vi "Control_Channel_Status.vi"() -> ()   [LabVIEW 2022 SP3]
uses:
  Sub VIs/ADAM Controls/Channel_State.ctl
  Sub VIs/ADAM Controls/Channel_names.ctl
  ADAM Server/ADAM_Global.vi
  Anemometry/Anemometry Sub Vis/Globals/Preference_global.vi
panel:
  out "Message":string
  out "List of Addresses":string[](array[string])
  in  "Address":u16(ring) items=["Show All", "0", "1", "502"]
  out "List of Ports":string[](array[string])
  in  "Port Names":u16(ring) items=["Show All", "", "LabVIEW", "10.244.4.15:502", "10.244.5.42"]
  out "Turn On?":bool
  in  "Turn Channel Off?":bool
  in  "stop":bool
  out "Ch State":T1
  in  "Turn Channels On?":bool
  in  "Selected Channels to Edit":i32[](listbox)
  in  "Search Charcters":string
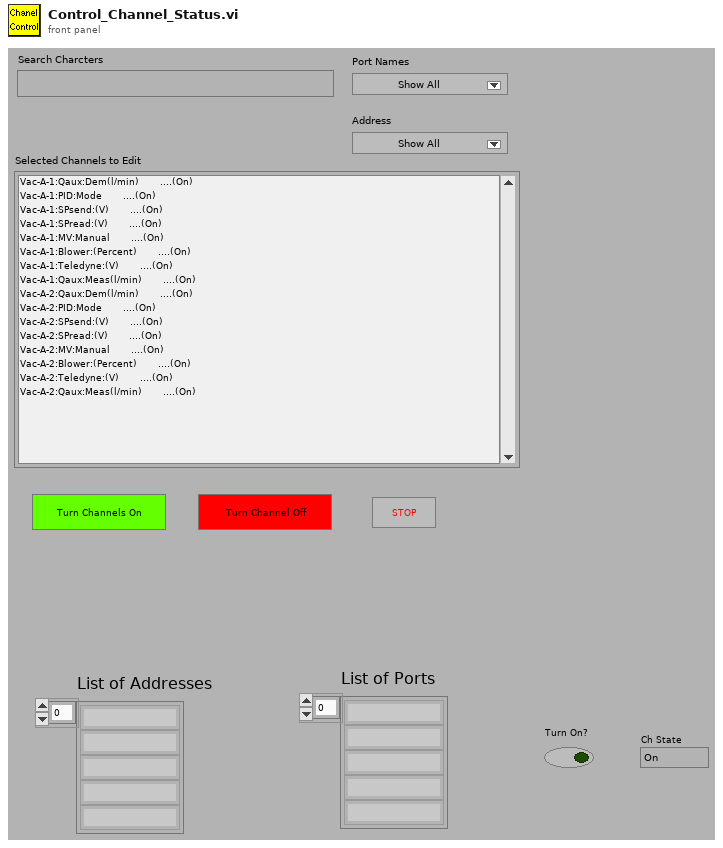
[diagram p1: front panel]
types:
  T1 = typedef "Channel_State.ctl" = enum16{"On", "Off", "Always On", "Always Off"}
  T2 = typedef "Channel_names.ctl" = enum16{"Active Only", "Active + Off", "All Channels", "Changeable Only", "Always Off", "Always On", "Always Off or On"}
  T3 = typedef "Server_Comms.ctl" = enum16{"Do Not Link To Server", "Server Link Healthy"}
  T4 = typedef "Ch_description_ADAM.ctl" = cluster{"Ch Name":string, "Type":T5, "Function":T6, "Ch State":T1, "Calibration type":T7, "A":dbl, "B":dbl, "C":dbl, "D":dbl, "Comments":string, "Address":T8, "String":string, "Duty":u16}
  T5 = typedef "Module_type_ADAM.ctl" = string
  T6 = typedef "Function_ADAM.ctl" = enum16{"Analogue Input", "Digital Input", "Event counter", "Event rate", "Analogue Output", "Digital Output", "Relay Output"}
  T7 = typedef "Calib_type_ADAM.ctl" = string
  T8 = typedef "Address.ctl" = cluster{"Main":i32, "Ch.":i32, "Sub":i32, "Port Name":string}
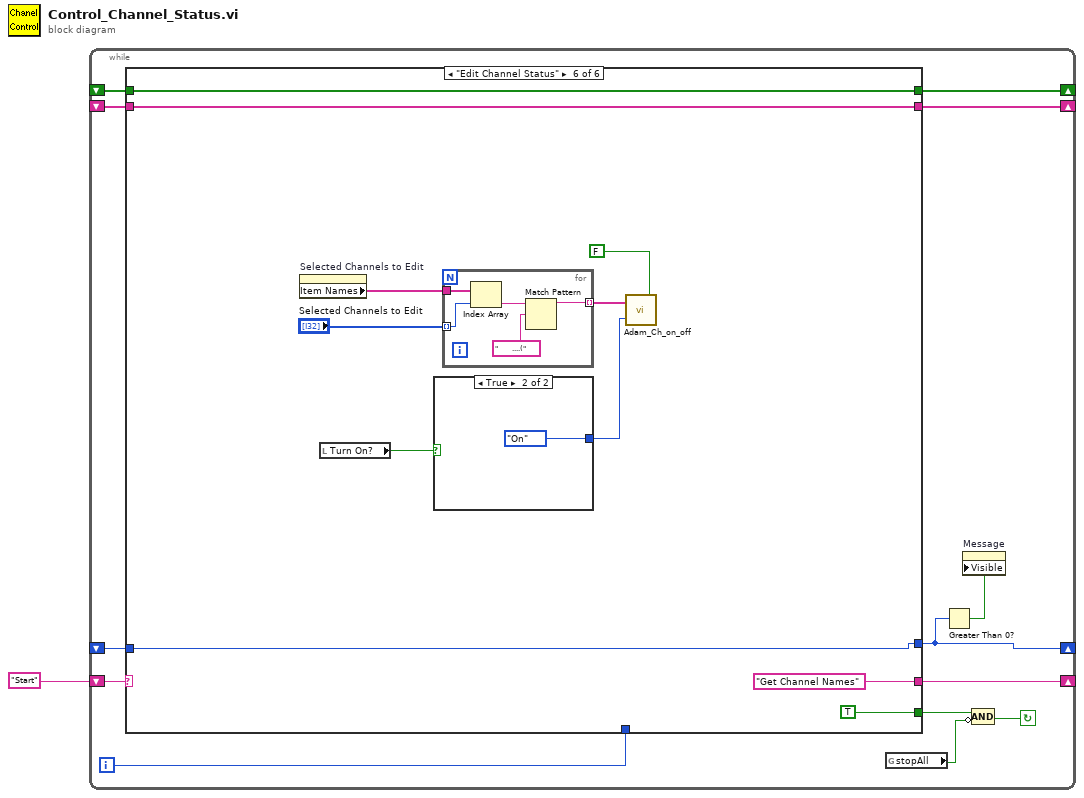
[diagram p0: block diagram]
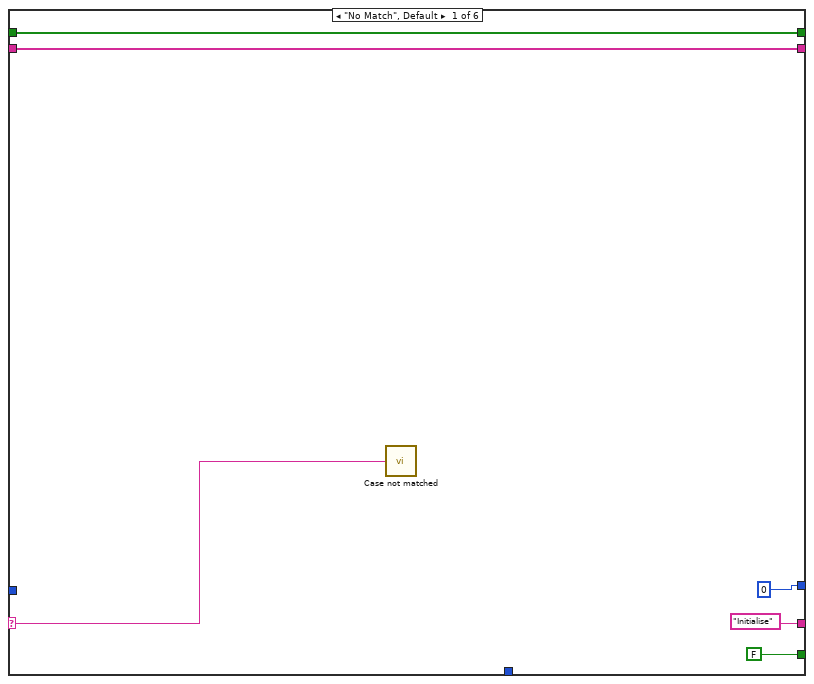
[diagram p2: hidden frame]
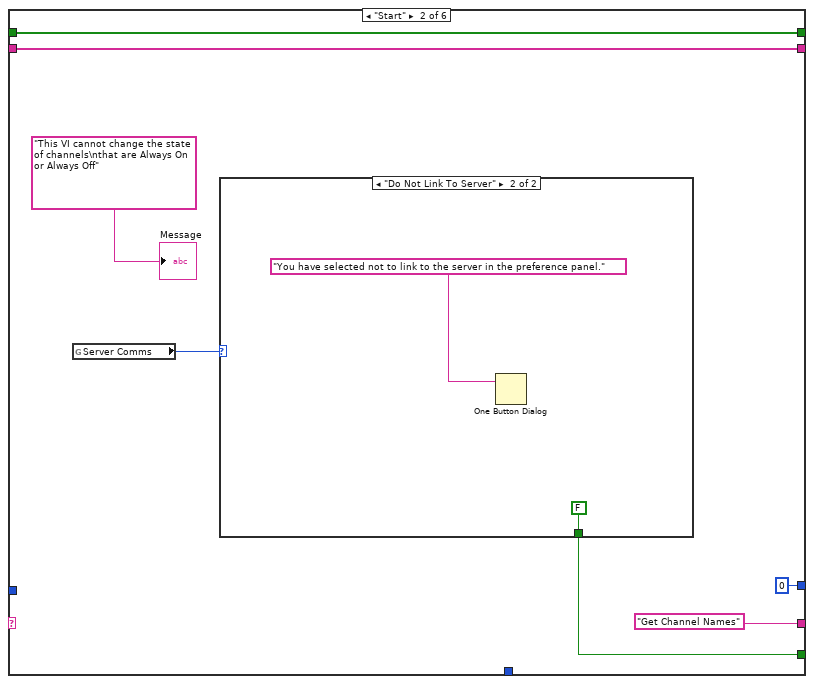
[diagram p3: hidden frame]
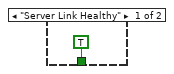
[diagram p4: hidden frame]
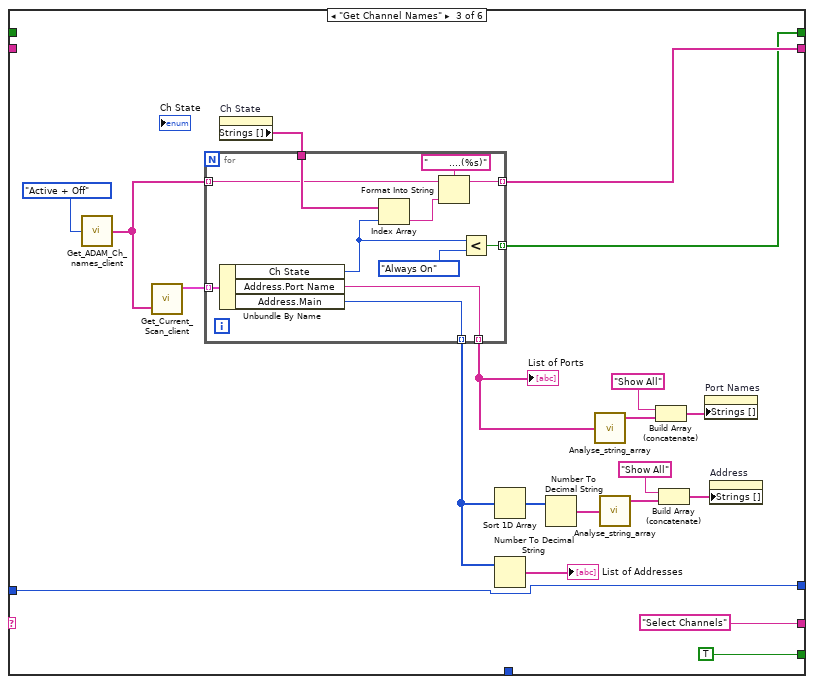
[diagram p5: hidden frame]
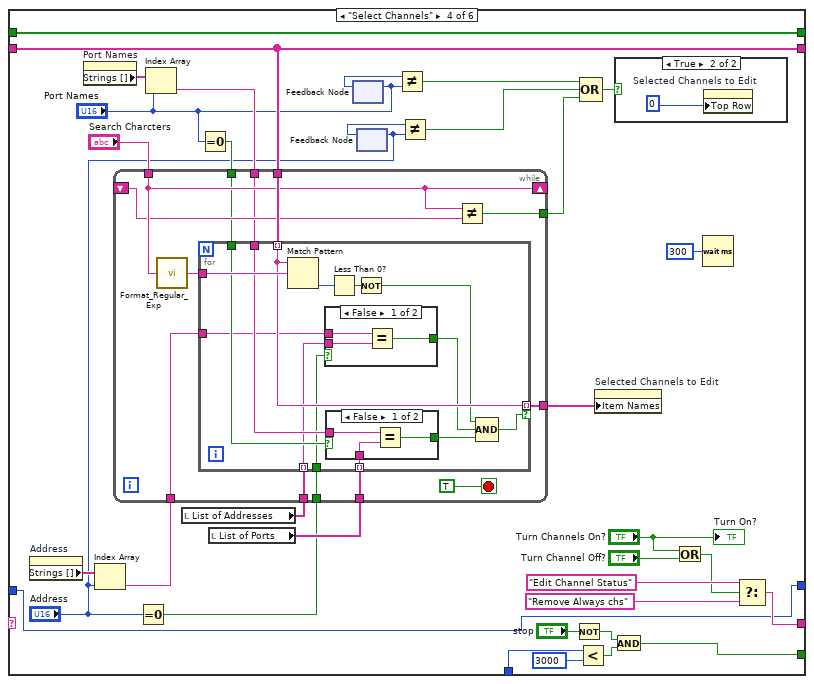
[diagram p6: hidden frame]
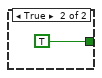
[diagram p8: hidden frame]
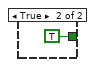
[diagram p9: hidden frame]
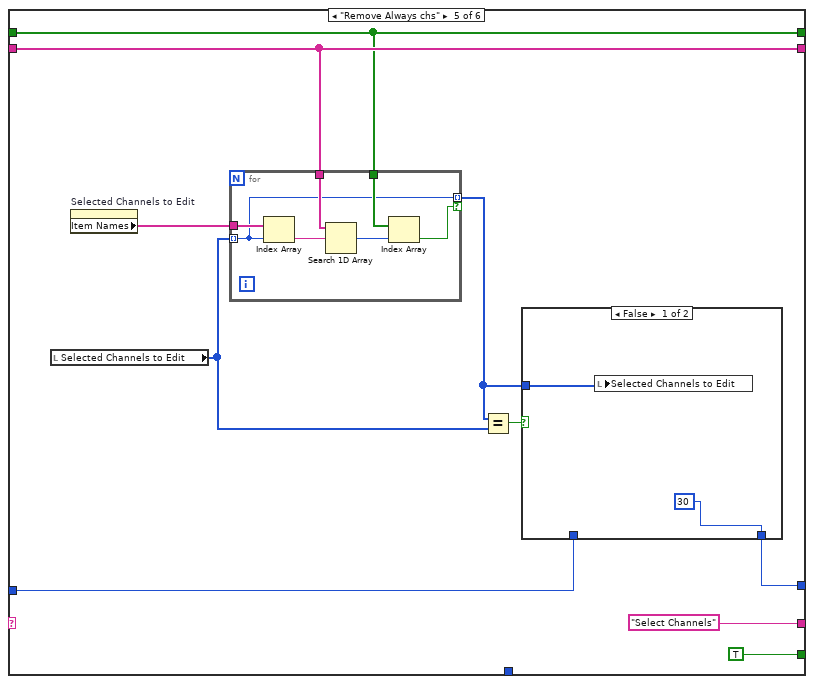
[diagram p10: hidden frame]
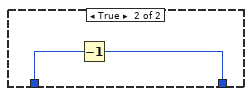
[diagram p11: hidden frame]
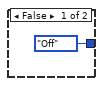
[diagram p12: hidden frame]
diagram:
  n1 = while {
    shift-left: "Start" -> [w13]
    shift-right: [w14] -> _
    shift-right: [w12] -> _
    shift-left: _ -> [w11]
    shift-right: [w9] -> _
    shift-left: _ -> [w8]
    shift-right: [w6] -> _
    shift-left: _ -> [w7]
    i -> [w10]
    stop <- w4 continue-if-true
    n2 = case shown="\"Edit Channel Status\"" w13 {
      selector: w13 -> [w16 _ _ _ _ _]
      tunnel: [FALSE w25 TRUE w82 TRUE TRUE] -> w3
      tunnel: ["Initialise" "Get Channel Names" "Select Channels" w92 "Select Channels" "Get Channel Names"] -> w14
      tunnel: [w18 w24 w44 w90 w138 w163] -> w12
      tunnel: w11 -> [w18 w24 _ w90 w138 w163]
      tunnel: w10 -> [_ _ _ w81 _ _]
      tunnel: [w17 w23 w32 w65 w137 w155] -> w9
      tunnel: w8 -> [w17 w23 _ w65 w137 w155]
      tunnel: [0 0 w31 w62 w133 w154] -> w6
      tunnel: w7 -> [_ _ w31 w62 w132 w154]
      frame "No Match", Default {
        n3 = call "Case not matched.vi"("Case Name not Matched"=w16) -> ()
      }
      frame "Start" {
        n4 = global read "Preference_global.vi" "Server Comms"() -> (w26:T3)
        n5 = case shown="\"Do Not Link To Server\"" w26 {
          tunnel: [TRUE FALSE] -> w25
          frame "Server Link Healthy" {
          }
          frame "Do Not Link To Server" {
            n6 = One Button Dialog(message="You have selected not to link to the server in the preference panel.") -> ()  [unwired: 2 out]
          }
        }
        "Message" <- "This VI cannot change the state of channels\nthat are Always On or Always Off"
      }
      frame "Get Channel Names" {
        n7 = call "Get_ADAM_Ch_names_client.vi"("Channel names set"=Channel_names."Active + Off") -> ("Ch names"=w45:string[])
        n8 = call "Get_Current_Scan_client.vi"("multipleChannels"=w45) -> ("Ch Description Array"=w47:T4[])  [unwired: 1 in, 3 out]
        n9 = property on="Ch State" class="Enum (strict)"() -> ("Strings []"=w46:string[])  [unwired: 2 in, 2 out]
        n10 = for {
          tunnel: w47 -> [w61] mode=indexing
          tunnel: w46 -> [w60]
          tunnel: w45 -> [w59] mode=indexing
          tunnel: [w56] -> w44 mode=indexing
          tunnel: [w55] -> w43 mode=indexing
          tunnel: [w54] -> w34 mode=indexing
          tunnel: [w51] -> w32 mode=indexing
          n11 = Unbundle By Name(w61) -> ("Ch State"=w53:T1, "Address.Port Name"=w55:string, "Address.Main"=w54:i32)
          n12 = Index Array(array=w60, index=w53) -> (element=w58:string)
          n13 = Format Into String(format string="       ....(%s)", initial string=w59, w58) -> (resulting string=w56:string)  [unwired: 1 in, 1 out]
          n14 = Less?(x=w53, y=Channel_State."Always On") -> (x < y?=w51:bool)
        }
        "List of Ports" <- w43
        n15 = Sort 1D Array(array=w34) -> (sorted array=w36:i32[])
        n16 = Number To Decimal String(number=w34) -> (decimal integer string=→"List of Addresses":string[])  [unwired: 1 in]
        n17 = Number To Decimal String(number=w36) -> (decimal integer string=w35:string[])  [unwired: 1 in]
        n18 = call "Analyse_string_array.vi"("String array"=w43) -> ("Unique strings"=w42:string[])  [unwired: 1 in, 1 out]
        n19 = call "Analyse_string_array.vi"("String array"=w35) -> ("Unique strings"=w38:string[])  [unwired: 1 in, 1 out]
        n20 = Build Array (concatenate)("Show All", w42) -> (w40:string[])
        n21 = Build Array (concatenate)("Show All", w38) -> (w37:string[])
        n22 = property on="Port Names" class="Ring (strict)"("Strings []"=w40) -> ()  [unwired: 2 in, 2 out]
        n23 = property on="Address" class="Ring (strict)"("Strings []"=w37) -> ()  [unwired: 2 in, 2 out]
      }
      frame "Select Channels" {
        n24 = property on="Address" class="Ring (strict)"() -> ("Strings []"=w74:string[])  [unwired: 2 in, 2 out]
        n25 = property on="Port Names" class="Ring (strict)"() -> ("Strings []"=w79:string[])  [unwired: 2 in, 2 out]
        n26 = Index Array(array=w74, index="Address") -> (element=w71:string)
        n27 = Equal To 0?(x="Address") -> (x = 0?=w70:bool)
        n28 = Index Array(array=w79, index="Port Names") -> (element=w78:string)
        n29 = local read "List of Addresses"() -> (w72:string[])
        n30 = Equal To 0?(x="Port Names") -> (x = 0?=w77:bool)
        n31 = local read "List of Ports"() -> (w73:string[])
        n32 = while {
          tunnel: [w103] -> w95
          tunnel: w90 -> [w109]
          tunnel: "Search Charcters" -> [w107]
          shift-right: [w107] -> _
          shift-left: _ -> [w106]
          tunnel: [w105] -> w63
          tunnel: w78 -> [w102]
          tunnel: w77 -> [w101]
          tunnel: w73 -> [w100]
          tunnel: w72 -> [w99]
          tunnel: w71 -> [w98]
          tunnel: w70 -> [w97]
          stop <- TRUE stop-if-true
          n33 = call "Format_Regular_Exp.vi"("Regular expression"=w107) -> ("Case Insensitive for html"=w108:string)
          n34 = for {
            tunnel: w108 -> [w123]
            tunnel: w109 -> [w121] mode=indexing
            tunnel: [w121] -> w103 mode=indexing if=w116
            tunnel: w102 -> [w118]
            tunnel: w100 -> [w119] mode=indexing
            tunnel: w101 -> [w115]
            tunnel: w99 -> [w114] mode=indexing
            tunnel: w98 -> [w113]
            tunnel: w97 -> [w112]
            n35 = Match Pattern(string=w121, regular expression=w123) -> (offset past match=w122:i32)  [unwired: 4 out]
            n36 = case shown="False" w112 {
              tunnel: w114 -> [w126 _]
              tunnel: w113 -> [w125 _]
              tunnel: [w124 TRUE] -> w110
              frame False {
                n37 = Equal?(x=w125, y=w126) -> (x = y?=w124:bool)
              }
              frame True {
              }
            }
            n38 = case shown="False" w115 {
              tunnel: w119 -> [w130 _]
              tunnel: w118 -> [w129 _]
              tunnel: [w128 TRUE] -> w117
              frame False {
                n39 = Equal?(x=w129, y=w130) -> (x = y?=w128:bool)
              }
              frame True {
              }
            }
            n40 = Less Than 0?(x=w122) -> (x < 0?=w120:bool)
            n41 = Not(x=w120) -> (.not. x?=w111:bool)
            n42 = Compound Arithmetic op=AND(w111, w110, w117) -> (w116:bool)
          }
          n43 = Not Equal?(x=w107, y=w106) -> (x != y?=w105:bool)
        }
        n44 = feedback-in #1("Port Names") -> ()
        n45 = feedback #1() -> (w76:u16)  [unwired: 1 in]
        n46 = feedback #2() -> (w69:u16)  [unwired: 1 in]
        n47 = feedback-in #2("Address") -> ()
        n48 = Not Equal?(x=w76, y="Port Names") -> (x != y?=w67:bool)
        n49 = Not Equal?(x=w69, y="Address") -> (x != y?=w64:bool)
        n50 = Not(x="stop") -> (.not. x?=w84:bool)
        n51 = Less?(x=w81, y=3000) -> (x < y?=w83:bool)
        n52 = Compound Arithmetic op=OR(w67, w64, w63) -> (w66:bool)
        n53 = property on="Selected Channels to Edit" class="LstBox (strict)"("Item Names"=w95) -> ()  [unwired: 2 in, 2 out]
        n54 = And(x=w84, y=w83) -> (x .and. y?=w82:bool)
        n55 = case shown="True" w66 {
          frame False {
          }
          frame True {
            n56 = property on="Selected Channels to Edit" class="LstBox (strict)"("Top Row"=0) -> ()  [unwired: 2 in, 2 out]
          }
        }
        n57 = Or(x="Turn Channels On?", y="Turn Channel Off?") -> (x .or. y?=w85:bool)
        n58 = Wait (ms)(milliseconds to wait=u32 300) -> ()  [unwired: 1 out]
        n59 = Select(t="Edit Channel Status", s=w85, f="Remove Always chs") -> (s? t:f=w92:string)
        "Turn On?" <- "Turn Channels On?"
      }
      frame "Remove Always chs" {
        n60 = local read "Selected Channels to Edit"() -> (w135:i32[])
        n61 = property on="Selected Channels to Edit" class="LstBox (strict)"() -> ("Item Names"=w139:string[])  [unwired: 2 in, 2 out]
        n62 = for {
          tunnel: w139 -> [w152]
          tunnel: w135 -> [w147] mode=indexing
          tunnel: w138 -> [w151]
          tunnel: w137 -> [w149]
          tunnel: [w147] -> w136 mode=indexing if=w146
          n63 = Index Array(array=w152, index=w147) -> (element=w150:string)
          n64 = Search 1D Array(1D array=w151, element=w150) -> (index of element=w148:i32)  [unwired: 1 in]
          n65 = Index Array(array=w149, index=w148) -> (element=w146:bool)
        }
        n66 = Equal?(x=w136, y=w135) -> (x = y?=w134:bool)
        n67 = case shown="False" w134 {
          tunnel: w136 -> [w143 _]
          tunnel: [30 w144] -> w133
          tunnel: w132 -> [_ w145]
          frame False {
            n68 = local write "Selected Channels to Edit"(w143) -> ()
          }
          frame True {
            n69 = Decrement(x=w145) -> (x-1=w144:i32)
          }
        }
      }
      frame "Edit Channel Status" {
        n70 = property on="Selected Channels to Edit" class="LstBox (strict)"() -> ("Item Names"=w159:string[])  [unwired: 2 in, 2 out]
        n71 = local read "Turn On?"() -> (w157:bool)
        n72 = case shown="True" w157 {
          tunnel: [Channel_State."Off" ("Ch State") Channel_State."On" ("Ch State")] -> w156
          frame False {
          }
          frame True {
          }
        }
        n73 = for {
          tunnel: "Selected Channels to Edit" -> [w170] mode=indexing
          tunnel: w159 -> [w169]
          tunnel: [w168] -> w158 mode=indexing
          n74 = Index Array(array=w169, index=w170) -> (element=w166:string)
          n75 = Match Pattern(string=w166, regular expression="       ....(" ("format string")) -> (before substring=w168:string)  [unwired: 4 out]
        }
        n76 = call "Adam_Ch_on_off.vi"("overrideAlwaysOn/Off? (T)"=FALSE, "desiredState"=w156, "ADAM Ch Names"=w158) -> ()
      }
    }
    n77 = global read "ADAM_Global.vi" "stopAll"() -> (w2:bool)
    n78 = Greater Than 0?(x=w6) -> (x > 0?=w5:bool)
    n79 = property on="Message" class="Str"("Visible"=w5) -> ()  [unwired: 2 in, 2 out]
    n80 = Compound Arithmetic op=AND(w3, invert w2) -> (w4:bool)
  }
